vi "FPGA_target_set_output.vi"(3 "tick_count_in":u32, 4 "data_in":T1, 6 "new_data_in":T1, 7 "set_outputs":bool=TRUE, 9 "C0_data":T2, 11 "C1_data":T2) -> (17 "tick_count_out":u32, 18 "data_out":T1)   [LabVIEW 2014]
doc: "writes a 64 bit pattern to the output lines"
uses:
  FPGA_32BitPattern_data_type.ctl
  FPGA_cmd_data_type.ctl
  <vilib>/rvi/eio/common/nirviEmuTemplateMethod_errors.vi
  <vilib>/eio/EIONode/EIONode.xnode
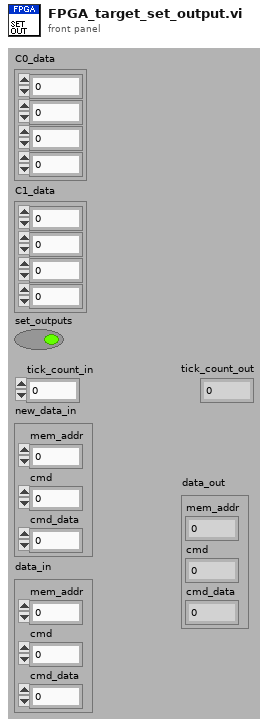
[diagram p1: front panel]
types:
  T1 = typedef "FPGA_cmd_data_type.ctl" = cluster{"mem_addr":u32, "cmd":u8, "cmd_data":u32}
  T2 = typedef "FPGA_32BitPattern_data_type.ctl" = cluster{"port0":u8, "port1":u8, "port2":u8, "port3":u8}
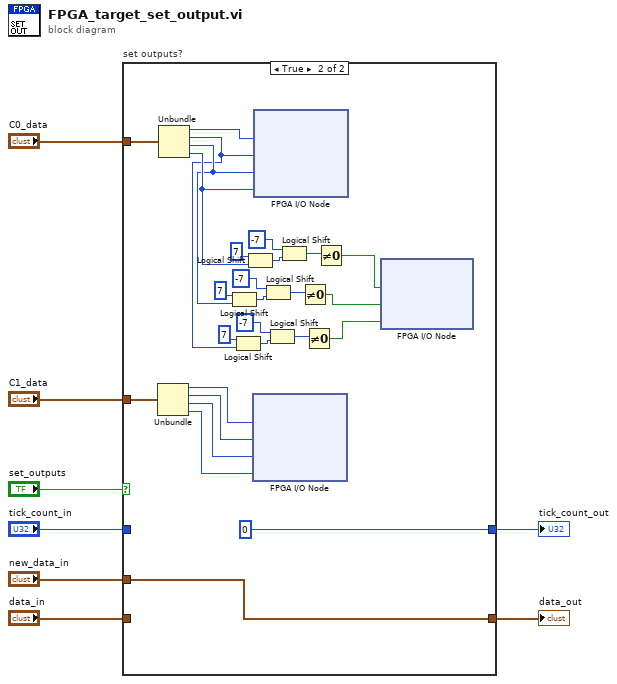
[diagram p0: block diagram]
diagram:
  n1 = case "set outputs?" shown="True" "set_outputs" {
    tunnel: [w10 u32 0] -> w8
    tunnel: "tick_count_in" -> [w10 _]
    tunnel: "C0_data" -> [_ w37]
    tunnel: "C1_data" -> [_ w31]
    tunnel: "new_data_in" -> [_ w29]
    tunnel: [w9 w29] -> w2
    tunnel: "data_in" -> [w9 _]
    frame False {
    }
    frame True {
      n2 = Unbundle(w31) -> ("port0"=w32:u8, "port1"=w33:u8, "port2"=w34:u8, "port3"=w35:u8)
      n3 = Unbundle(w37) -> ("port0"=w36:u8, "port1"=w12:u8, "port2"=w18:u8, "port3"=w25:u8)
      n4 = Logical Shift(y=i16 7, x=w18) -> (x << y=w21:u8)
      n5 = Logical Shift(y=i16 7, x=w12) -> (x << y=w15:u8)
      n6 = Logical Shift(y=i16 7, x=w25) -> (x << y=w27:u8)
      n7 = xnode ("FPGA I/O Node")("DO_56-63"=w32, "DO_48-55"=w33, "DO_40-47"=w34, "DO_32-39"=w35) -> ()  [unwired: 4 in, 4 out]
      n8 = xnode ("FPGA I/O Node")("DO_24-31"=w36, "DO_16-23"=w12, "DO_08-15"=w18, "DO_00-07"=w25) -> ()  [unwired: 4 in, 4 out]
      n9 = Logical Shift(y=i16 -7, x=w21) -> (x << y=w19:u8)
      n10 = Logical Shift(y=i16 -7, x=w15) -> (x << y=w13:u8)
      n11 = Logical Shift(y=i16 -7, x=w27) -> (x << y=w24:u8)
      n12 = Not Equal To 0?(x=w19) -> (x != 0?=w17:bool)
      n13 = Not Equal To 0?(x=w13) -> (x != 0?=w11:bool)
      n14 = Not Equal To 0?(x=w24) -> (x != 0?=w23:bool)
      n15 = xnode "FPGA I/O Node"("PXI_Trig0"=w23, "PXI_Trig1"=w17, "PXI_Trig2"=w11) -> ()  [unwired: 3 in, 3 out]
    }
  }
  "tick_count_out" <- w8
  "data_out" <- w2
